vi "Test_Get_Angle_And_Dist_To_Speaker.vi"() -> ()   [LabVIEW 2023]
uses:
  GeneralPurpose/AllianceColorGlobal.vi
  Vision/VisionGlobal.vi
  <vilib>/Rock Robotics/WPI/ThirdParty/JAS_Junk/TrajLib/Trajectory_Library.lvlib
  <vilib>/Rock Robotics/WPI/DriverStation/WPI_DriverStationAllianceInfo.ctl
  <vilib>/Rock Robotics/WPI/ThirdParty/JAS_Junk/TrajLib/TypeDef/FieldDisp_ElementPicture.ctl
panel:
  out "OnTarget":bool
  out "lAngle 1":dbl
  out "Change":dbl
  out "Angle":dbl
  out "DesiredSpeed (degree/s)":dbl
  out "ROBOT":T1
  out "Field Picture":picture
  in  "X":dbl step=0.1
  in  "Y":dbl step=0.1
  in  "Alliance":T2
  out "AngleDegrees":dbl
  out "Distance":dbl
  # "Robot Position\nMeters"
  # "Meters"
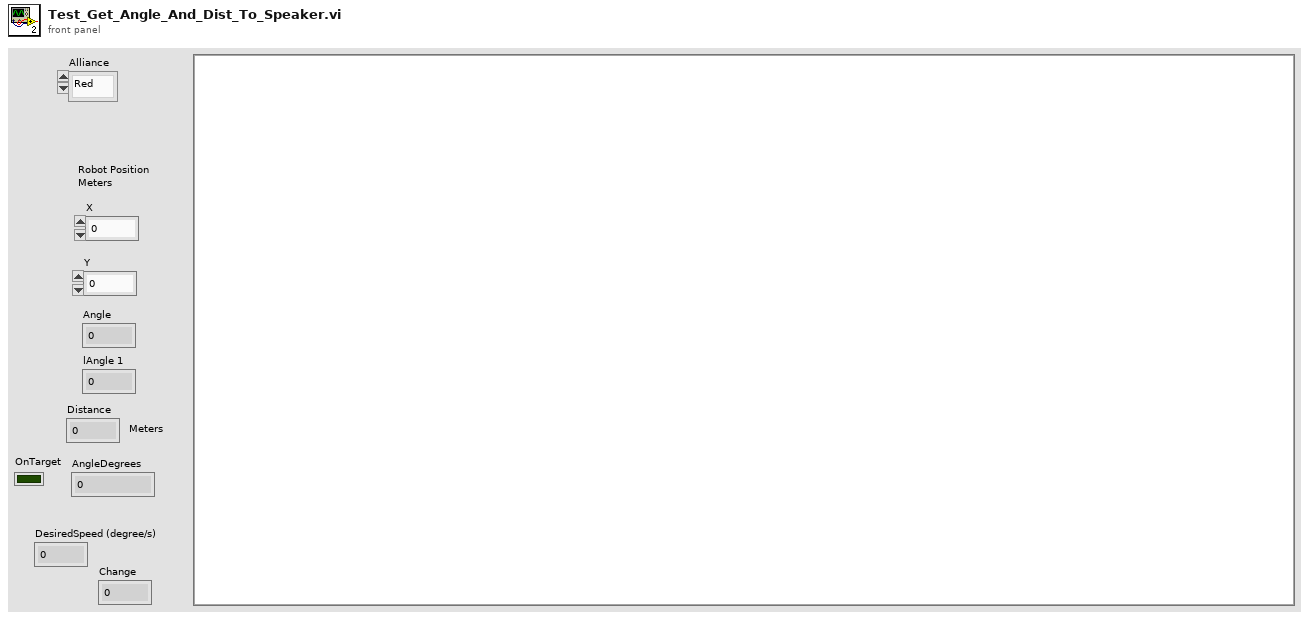
[diagram p1: front panel]
types:
  T1 = typedef "Trajectory_Library.lvlib/FieldDisp_ElementPicture.ctl" = picture
  T2 = typedef "WPI_DriverStationAllianceInfo.ctl" = enum16{"Red", "Blue", "Invalid"}
  T3 = typedef "Trajectory_Library.lvlib/FieldDisp_FieldElement.ctl" = cluster{"ONE-8-bit pixmap":u8[][], "Two-Array":cdb[][], "Three-Numeric":i32, "Four-Numeric":i32, "Five-Numeric":cdb, "Six-colors":u32[], "Seven-new element/subarray":u32, "Left Pixel":dbl, "Top Pixel":dbl, "Width Pix/Ft":dbl, "Height Pix/Ft":dbl, "Element Picture Ref":refnum<vi>}
  T4 = typedef "Trajectory_Library.lvlib/POSE2D.ctl" = cluster{"TRANSLATION":T5, "ROTATION":T6}
  T5 = typedef "Trajectory_Library.lvlib/TRANSLATION2D.ctl" = cluster{"X":dbl, "Y":dbl}
  T6 = typedef "Trajectory_Library.lvlib/ROTATION2D.ctl" = cluster{"VALUE":dbl, "COS":dbl, "SIN":dbl}
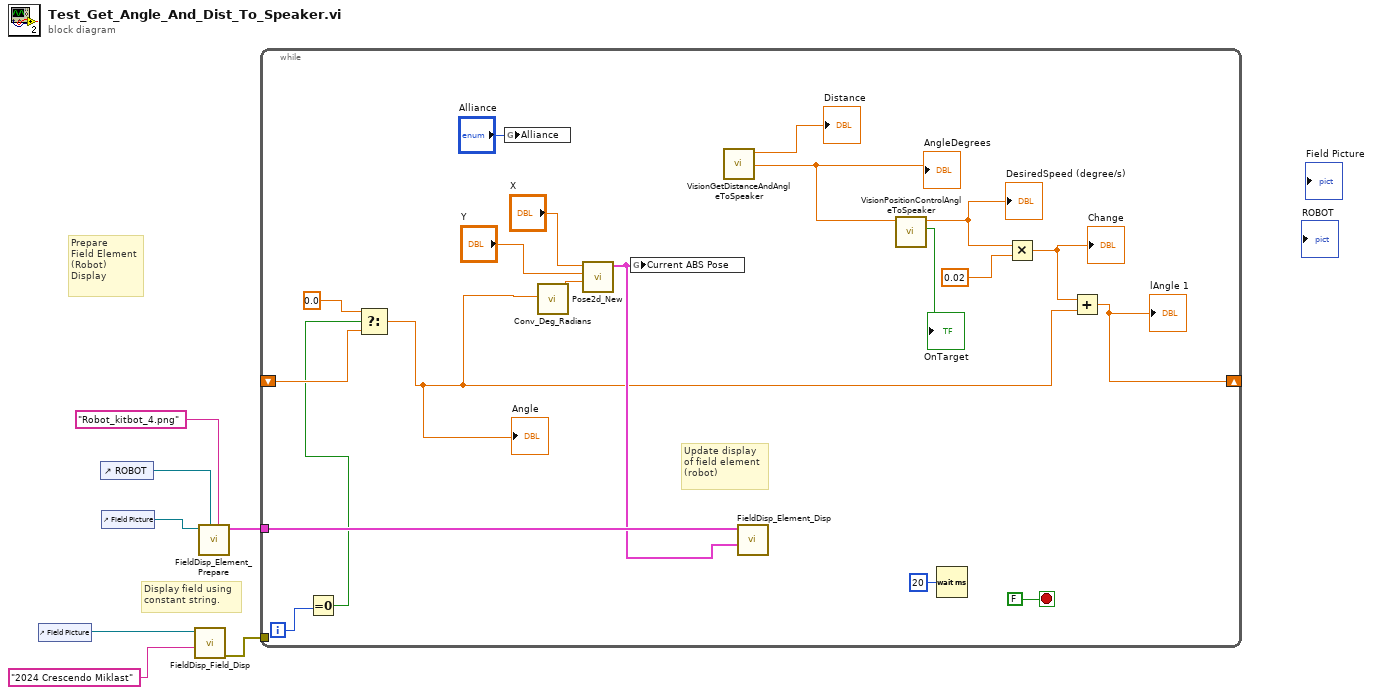
[diagram p0: block diagram]
diagram:
  # "Prepare\nField Element\n(Robot)\nDisplay"
  # "Display field using\nconstant string."
  n1 = control-ref of="Field Picture"() -> (w5:refnum<vi>)
  n2 = control-ref of="ROBOT"() -> (w6:refnum<vi>)
  n3 = control-ref of="Field Picture"() -> (w7:refnum<vi>)
  n4 = call <vilib>:"FieldDisp_Field_Disp.vi"("Field Selector"="2024 Crescendo Miklast", "Picture in"=w5) -> ("error out"=w1:errorcluster)  [unwired: 9 in]
  n5 = call <vilib>:"FieldDisp_Element_Prepare.vi"("Element File Name"="Robot_kitbot_4.png" ("Picture FIle Name"), "Element Picture Ref"=w6, "Field Picture Ref"=w7) -> ("Field Element Info"=w2:T3)  [unwired: 7 in, 1 out]
  n6 = while {
    tunnel: w2 -> [w20]
    tunnel: w1 -> [_]
    shift-right: [w12] -> _
    shift-left: _ -> [w11]
    i -> [w10]
    stop <- FALSE stop-if-true
    # "Update display\nof field element\n(robot)"
    n7 = Equal To 0?(x=w10) -> (x = 0?=w9:bool)
    n8 = Select(t=0.0, s=w9, f=w11) -> (s? t:f=w13:dbl)
    "Angle" <- w13
    n9 = global write "AllianceColorGlobal.vi" "Alliance"("Alliance") -> ()
    n10 = call <vilib>:"Conv_Deg_Radians.vi"("Degress"=w13) -> ("Radians"=w23:dbl)  [unwired: 10 in]
    n11 = call <vilib>:"Pose2d_New.vi"("Heading"=w23, "Y"="Y", "X"="X") -> ("out POSe"=w19:T4)  [unwired: 8 in]
    n12 = global write "VisionGlobal.vi" "Current ABS Pose"(w19) -> ()
    n13 = call "VisionGetDistanceAndAngleToSpeaker.vi"() -> ("DesiredAngle"=w18:dbl, "Distance"=→"Distance":dbl)  [unwired: 10 in]
    "AngleDegrees" <- w18
    n14 = call <vilib>:"FieldDisp_Element_Disp.vi"("Element Pose"=w19, "Element Info"=w20) -> ()  [unwired: 10 in]
    n15 = call "VisionPositionControlAngleToSpeaker.vi"("TargetAngle"=w18) -> ("OnTargetSpeaker"=→"OnTarget":bool, "DesiredAngularSpeed (degree/s)"=w17:dbl)  [unwired: 9 in]
    "DesiredSpeed (degree/s)" <- w17
    n16 = Wait (ms)(milliseconds to wait=u32 20) -> ()  [unwired: 1 out]
    n17 = Multiply(x=w17, y=0.02) -> (x*y=w15:dbl)
    "Change" <- w15
    n18 = Add(x=w15, y=w13) -> (x+y=w12:dbl)
    "lAngle 1" <- w12
  }
